vi "deinitialize.vi"(0 "HGF_ImaqDx":refnum<class "HGF_ImaqDx.lvclass">, 5 "error in (no error)":errorcluster) -> (19 "error out":errorcluster)   [LabVIEW 2014, in "HGF_IMAQ.lvlib" / "HGF_ImaqDx.lvclass"]
doc: "This is a dynamic dispatch VI. It can be overwritten by childclasses to release allocated recources."
uses:
  HGF_ImaqDx.lvclass
  HGF_IMAQDevice/HGF_IMAQDevice.lvclass
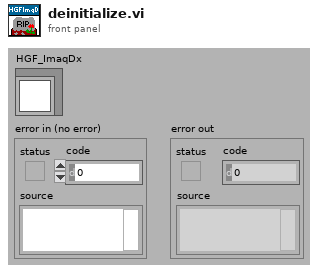
[diagram p1: front panel]
types:
  T1 = typedef "IMAQdx.ctl" = refnum<k21>
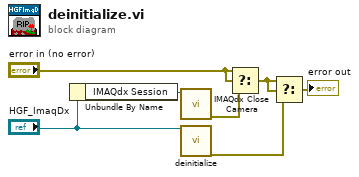
[diagram p0: block diagram]
diagram:
  n1 = Unbundle By Name("HGF_ImaqDx") -> ("IMAQdx Session"=w2:T1)
  n2 = call <vilib>:"IMAQdx Close Camera.vi"("Session In"=w2) -> ("error out"=w1:errorcluster)  [unwired: 1 in, 9 out]
  n3 = call-parent "deinitialize.vi"("HGF_IMAQDevice"="HGF_ImaqDx") -> ("error out"=w4:errorcluster)  [unwired: 1 in, 17 out]
  n4 = Select(t="error in (no error)", s="error in (no error)", f=w1) -> (s? t:f=w5:errorcluster)
  n5 = Select(t=w5, s=w5, f=w4) -> (s? t:f=→"error out":errorcluster)
